vi "setXmlNode.vi"(8 "error in (no error)":errorcluster, 10 "xmlNode":refnum<class "xmlNode.lvclass">, 11 "Channel.lvclass in":refnum<class "Channel.lvclass">) -> (0 "error out":errorcluster, 3 "Channel.lvclass out":refnum<class "Channel.lvclass">)   [LabVIEW 2009, in "Tools.lvlib" / "DatabaseHelpers.lvlib" / "Channel.lvclass"]
uses:
  Channel.lvclass
  xmlNode/xmlNode.lvclass
  Channel.lvclass/Channel.ctl
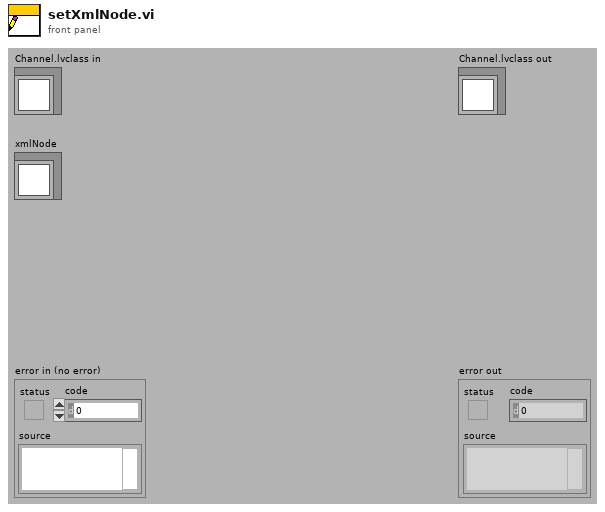
[diagram p1: front panel]
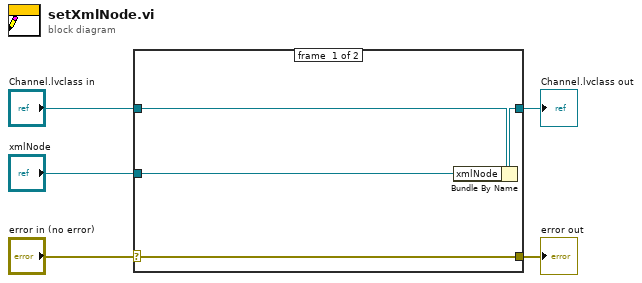
[diagram p0: block diagram]
diagram:
  n1 = case shown="No Error" "error in (no error)" {
    selector: "error in (no error)" -> [w9 w10]
    tunnel: [w9 w10] -> w4
    tunnel: [w7 w11] -> w2
    tunnel: "Channel.lvclass in" -> [w8 w11]
    tunnel: "xmlNode" -> [w6 _]
    frame #0 {
      n2 = Bundle By Name(cluster=w8, "xmlNode"=w6) -> (w7:refnum<class "Channel.lvclass">)
    }
    frame #1 {
    }
  }
  "error out" <- w4
  "Channel.lvclass out" <- w2
